vi "BuildConcentrationString.vi"(1 "Concentrations":dbl[](array[numeric])) -> (0 "Concentration String":string[](array[string]))   [LabVIEW 2013]
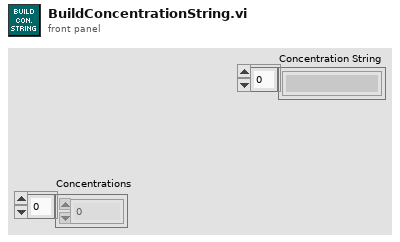
[diagram p1: front panel]
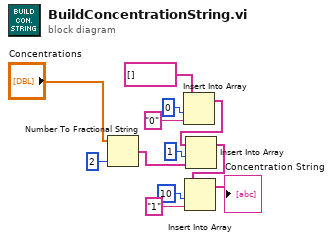
[diagram p0: block diagram]
diagram:
  n1 = Number To Fractional String(number="Concentrations", precision (6)=i16 2) -> (F-format string=w5:string[])  [unwired: 2 in]
  n2 = Insert Into Array(array=string[] [], index=0, new element="0" ("new element/subarray")) -> (w6:string[])
  n3 = Insert Into Array(array=w6, index=1, new element=w5) -> (w2:string[])
  n4 = Insert Into Array(array=w2, index=10, new element="1" ("new element/subarray")) -> (→"Concentration String":string[])
